vi "Reload Bitfile.vi"(7 "Group":bool, 8 "error in (no error)":errorcluster, 10 "NewVal":path, 11 "Item Ref in":T1 format="%.0x") -> (0 "error out":errorcluster, 3 "Section Ref out":T1 format="%.0x")   [LabVIEW 2018, in "FPGA Addon System Explorer.lvlib"]
uses:
  FPGA Addon System Explorer.lvlib
  <vilib>/NI Veristand/Custom Device API/Custom Device Item Ref.ctl
  Addon Shared/SubVIs/Constants.vi
  Addon Shared/FPGA Addon Shared.lvlib
  <vilib>/NI Veristand/Custom Device API/Custom Device API.lvlib
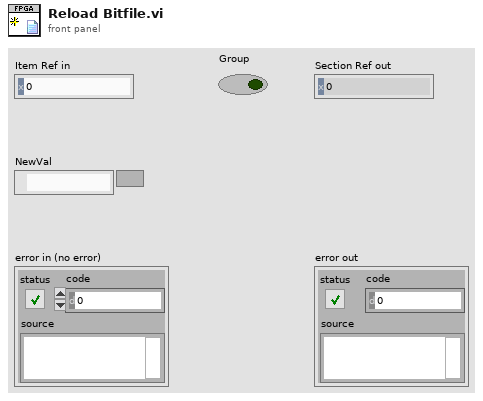
[diagram p1: front panel]
types:
  T1 = typedef "Custom Device API.lvlib/Custom Device Item Ref.ctl" = u64
  T2 = typedef "Fifo_DMA_Config.ctl" = cluster{"Name":string, "Depth":u32, "Write? (Deprecated:Use Implementation)":bool, "Physical Channel":u32, "Base Address":u32, "Data Width":u32, "Data Type":T3, "FXP Properties":variant, "Write Window Address":u32, "Implementation":T4, "Control Set":u32}
  T3 = typedef "niFpgaDataTypeControl.ctl" = enum32{"Boolean", "I8", "I16", "I32", "I64", "U8", "U16", "U32", "U64", "FXP", "CustomControl", "SGL"}
  T4 = typedef "niFpgaDmaChannelImplementation.ctl" = enum16{"niFpgaTargetToHost", "niFpgaHostToTarget", "niFpgaPeerToPeerWriter", "niFpgaPeerToPeerReader", "niCoreTargetToHost", "niCoreHostToTarget"}
  T5 = typedef "niFpgaBitfileStructure_VI.ctl" = cluster{"Name":string, "RegisterMap":T6[], "Icon":T11}
  T6 = typedef "nirviControlStructure.ctl" = cluster{"Name":string, "Hidden":bool, "Indicator":bool, "Flattened Type":string, "Grouping":cluster{"Grouped":bool, "Member Names":string[], "Member IDs":u32[]}, "Address":u32, "Size":u32, "Class":u32, "Internal":bool, "Typedef":T7, "ID":u32, "Bidirectional":bool, "Synchronous":bool, "Mechanical Action":T8, "Sub Controls":T9[], "Access May Timeout":bool, "Register Node":bool}
  T7 = typedef "nirviTypdefDescription.ctl" = cluster{"Typedef":bool, "Path":path}
  T8 = typedef "nirviMechanicalAction.ctl" = enum8{"Switch When Pressed", "Switch When Released", "Switch Until Released", "Latch When Pressed", "Latch When Released", "Latch Until Released"}
  T9 = typedef "nirviSubControlStructure.ctl" = cluster{"Name":string, "flattened Type":string, "Cluster Information":T10, "Typedef":T7}
  T10 = typedef "nirviClusterElementControl.ctl" = cluster{"Name Hierarchy":string[], "Item Order":u32[]}
  T11 = typedef "imagedata.ctl" = cluster{"image type":i32, "image depth":i32, "image":u8[], "mask":u8[], "colors":u32[], "Rectangle":cluster{"left":i16, "top":i16, "right":i16, "bottom":i16}}
  T12 = typedef "FPGA Addon Shared.lvlib/Register Information.ctl" = cluster{"Name":string, "Data Type":T13, "Default Value":variant}
  T13 = typedef "FPGA Addon Shared.lvlib/Data Type.ctl" = enum8{"<Null>", "I8", "I16", "I32", "I64", "U8", "U16", "U32", "U64", "SGL", "Boolean", "Analog PWM In Settings", "Analog PWM In", "Digital PWM In Settings", "Digital PWM In", "Digital PWM Out", "Sine Out", "FXP+/-24.5", "FXP+/-16.5", "FXP+/-32.8", "FXP+/-64.32", "FXP+/-16.7", "FXP+/-20.5", "FXP+/-27.5", "FXP+/-32.16", "FXP+16.3", "FXP+18.3", "Digital Static In", "Digital Static Out", "Digital Static In Settings", "Digital WSS Out", "Quad Encoder Settings", "Quad Encoder In", "Group"}
  T14 = typedef "FPGA Addon Shared.lvlib/DMA Information.ctl" = cluster{"Name":string, "Data Type":T13}
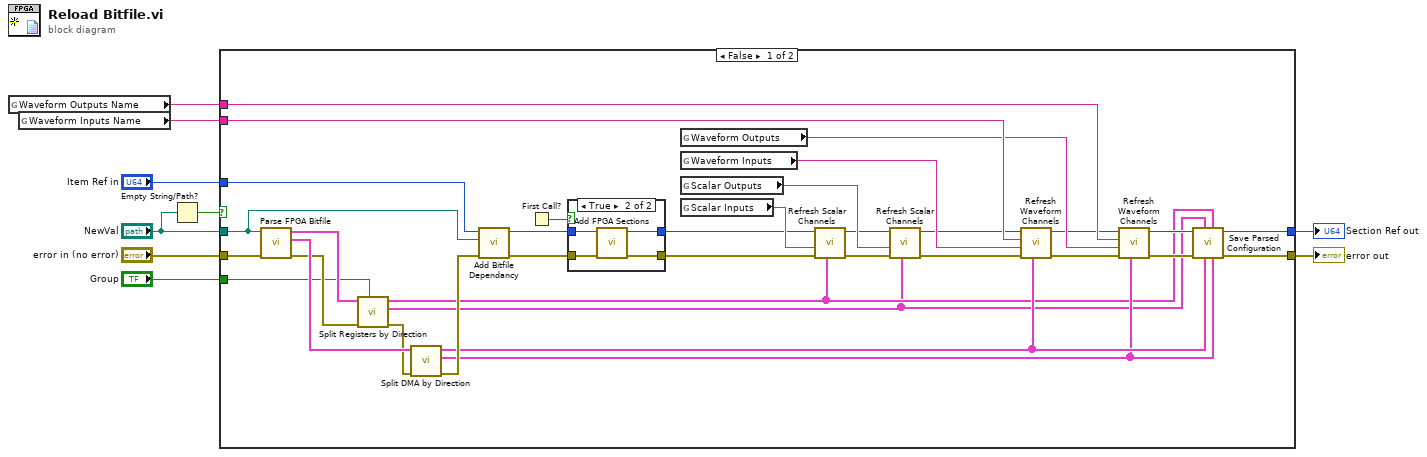
[diagram p0: block diagram]
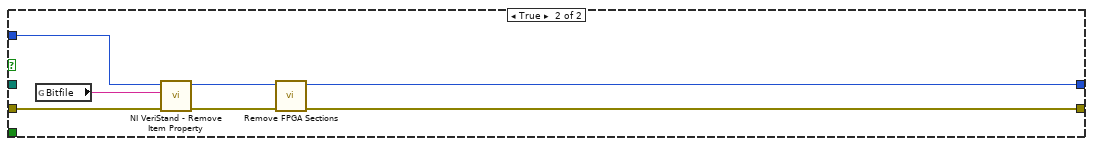
[diagram p3: hidden frame]
diagram:
  n1 = global read "Constants.vi" "Waveform Outputs Name"() -> (w8:string)
  n2 = global read "Constants.vi" "Waveform Inputs Name"() -> (w9:string)
  n3 = Empty String/Path?(string/path="NewVal") -> (empty?=w5:bool)
  n4 = case shown="False" w5 {
    tunnel: "NewVal" -> [w38 _]
    tunnel: "error in (no error)" -> [w43 w51]
    tunnel: w9 -> [w25 _]
    tunnel: w8 -> [w21 _]
    tunnel: [w40 w56] -> w7
    tunnel: [w39 w55] -> w6
    tunnel: "Item Ref in" -> [w37 w53]
    tunnel: "Group" -> [w12 _]
    frame False {
      n5 = call "Parse FPGA Bitfile.vi"("error in (no error)"=w43, "Path"=w38) -> ("error out"=w36:errorcluster, "DMA configuration array"=w42:T2[], "vi info"=w41:T5)  [unwired: 7 in]
      n6 = call "Split Registers by Direction.vi"("Group"=w12, "error in"=w36, "vi info"=w41) -> ("error out"=w35:errorcluster, "Controls"=w10:T12[], "Indicator"=w11:T12[])  [unwired: 6 in]
      n7 = call "Split DMA by Direction.vi"("error in"=w35, "DMA configuration array"=w42) -> ("error out"=w34:errorcluster, "HostToTarget"=w17:T14[], "TargetToHost"=w23:T14[])  [unwired: 7 in]
      n8 = call "Add Bitfile Dependancy.vi"("error in (no error)"=w34, "Path"=w38, "Item Ref in"=w37) -> ("error out"=w32:errorcluster, "Item Ref out"=w33:T1)  [unwired: 7 in]
      n9 = First Call?() -> (First Call?: T/F=w30:bool)
      n10 = case shown="True" w30 {
        tunnel: w33 -> [w45 w49]
        tunnel: w32 -> [w44 w48]
        tunnel: [w44 w47] -> w31
        tunnel: [w45 w46] -> w14
        frame False {
        }
        frame True {
          n11 = call "Add FPGA Sections.vi"("error in (no error)"=w48, "Node Ptr"=w49) -> ("error out"=w47:errorcluster, "Parent Ref out"=w46:T1)  [unwired: 8 in]
        }
      }
      n12 = global read "Constants.vi" "Waveform Outputs"() -> (w22:string)
      n13 = global read "Constants.vi" "Waveform Inputs"() -> (w26:string)
      n14 = global read "Constants.vi" "Scalar Outputs"() -> (w28:string)
      n15 = global read "Constants.vi" "Scalar Inputs"() -> (w15:string)
      n16 = call "Refresh Scalar Channels.vi"("scalar channels"=w11, "error in (no error)"=w31, "scalar type GUID"=w15, "scalar section ref in"=w14) -> ("error out"=w29:errorcluster, "scalar section ref out"=w13:T1)  [unwired: 6 in]
      n17 = call "Refresh Scalar Channels.vi"("scalar channels"=w10, "error in (no error)"=w29, "scalar type GUID"=w28, "scalar section ref in"=w13) -> ("error out"=w27:errorcluster, "scalar section ref out"=w24:T1)  [unwired: 6 in]
      n18 = call "Refresh Waveform Channels.vi"("new bitfile dma channels"=w23, "error in (no error)"=w27, "waveform type GUID"=w26, "waveform inputs name"=w25, "item ref in"=w24) -> ("error out"=w19:errorcluster, "item ref out"=w20:T1)  [unwired: 5 in]
      n19 = call "Refresh Waveform Channels.vi"("new bitfile dma channels"=w17, "error in (no error)"=w19, "waveform type GUID"=w22, "waveform inputs name"=w21, "item ref in"=w20) -> ("error out"=w18:errorcluster, "item ref out"=w16:T1)  [unwired: 5 in]
      n20 = call "Save Parsed Configuration.vi"("HostToTarget DMAs"=w17, "Indicators"=w11, "TargetToHost DMAs"=w23, "Controls"=w10, "error in (no error)"=w18, "Parent Ref in"=w16) -> ("error out"=w40:errorcluster, "Section Ref out"=w39:T1)  [unwired: 4 in]
    }
    frame True {
      n21 = global read "Constants.vi" "Bitfile"() -> (w54:string)
      n22 = call <vilib>:"NI VeriStand - Remove Item Property.vi"("error in (no error)"=w51, "Property Name"=w54, "Item Ref in"=w53) -> ("error out"=w50:errorcluster, "Item Ref out"=w52:T1)  [unwired: 6 in, 1 out]
      n23 = call "Remove FPGA Sections.vi"("error in (no error)"=w50, "Item Ref in"=w52) -> ("error out"=w56:errorcluster, "Item Ref out"=w55:T1)  [unwired: 8 in]
    }
  }
  "error out" <- w7
  "Section Ref out" <- w6
